vi "Get VI Tester Reference.vi"(8 "error in":errorcluster, 11 "application reference (This Application)":refnum<vi>) -> (0 "error out":errorcluster, 2 "vi reference":refnum<vi>)   [LabVIEW 2011, in "VI Tester Project API.lvlib"]
uses:
  VI Tester Project API.lvlib
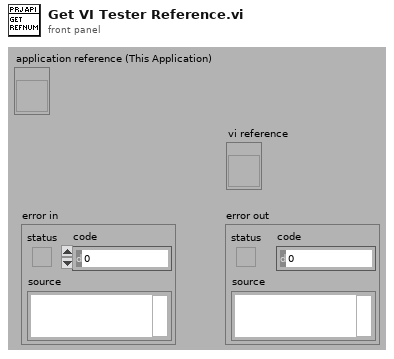
[diagram p1: front panel]
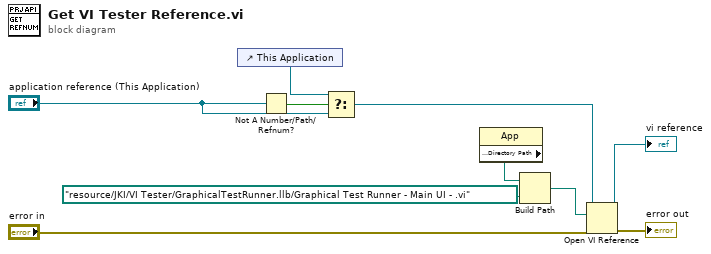
[diagram p0: block diagram]
diagram:
  n1 = control-ref of="This Application"() -> (w4:refnum<vi>)
  n2 = Not A Number/Path/Refnum?(number/path/refnum="application reference (This Application)") -> (NaN/Path/Refnum?=w5:bool)
  n3 = Select(t=w4, s=w5, f="application reference (This Application)") -> (s? t:f=w2:refnum<vi>)
  n4 = property class="App"() -> ("Application:Directory Path"=w7:path)  [unwired: 2 in, 2 out]
  n5 = Build Path(base path=w7, name or relative path=path "resource/JKI/VI Tester/GraphicalTestRunner.llb/Graphical Test Runner - Main UI - .vi" ("path")) -> (appended path=w1:path)
  n6 = Open VI Reference(application reference (local)=w2, vi path=w1, error in (no error)="error in") -> (vi reference=→"vi reference":refnum<vi>, error out=→"error out":errorcluster)  [unwired: 3 in]
